vi "get_saved_XYZ_pos.vi"(11 "MotorSystem.lvclass input":refnum<class "MotorSystem.lvclass">) -> (2 "points":cluster{"X":dbl, "Y":dbl, "Z":dbl}[](array[cluster]), 3 "MotorSystem.lvclass output":refnum<class "MotorSystem.lvclass">)   [LabVIEW 2016, in "MotionControl_UFO_3DOF.lvlib" / "MotorSystem.lvclass"]
uses:
  <userlib>/MotionControl_UFO_3DOF/MotorSystem/MotorSystem.lvclass
  <userlib>/MotionControl_UFO_3DOF/MotorSystem/MotorSystem.lvclass/MotorSystem.ctl
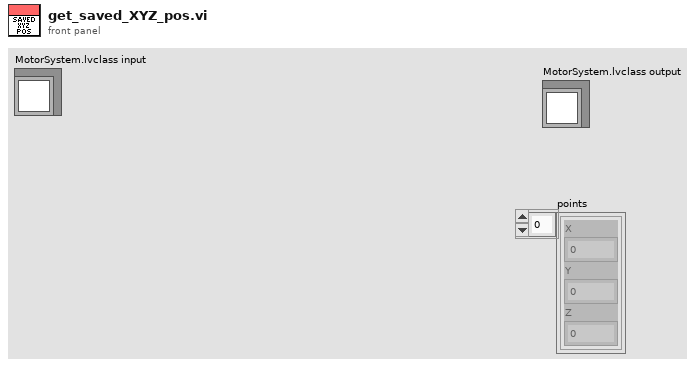
[diagram p1: front panel]
types:
  T1 = typedef "MotionControl_UFO_3DOF.lvlib/MotorSystem.lvclass/SavedPosCluster.ctl" = cluster{"name":string, "command list":T2}
  T2 = typedef "MotionControl_UFO_3DOF.lvlib/MotorSystem.lvclass/CommandList.ctl" = cluster{"cmd":T3, "cmd info":T4[]}[]
  T3 = typedef "MotionControl_UFO_3DOF.lvlib/MotorSystem.lvclass/cmd_system.ctl" = enum16{"NONE", "MOVE_SYSTEM", "WAIT_UNTIL_MOVE_DONE", "EXIT", "WAIT_UNTIL_SELECTED_MOVE_DONE", "WAIT_A_TIME"}
  T4 = typedef "MotionControl_UFO_3DOF.lvlib/MotorSystem.lvclass/SavedDimensionCluster.ctl" = cluster{"dimension name":string, "pos":dbl, "unit mode":T5, "unit conversion ratio":dbl}
  T5 = typedef "MotionControl_UFO_3DOF.lvlib/OneMotion.lvclass/unit mode.ctl" = enum16{"motor (pulse)", "linear (mm) or radial (degree)"}
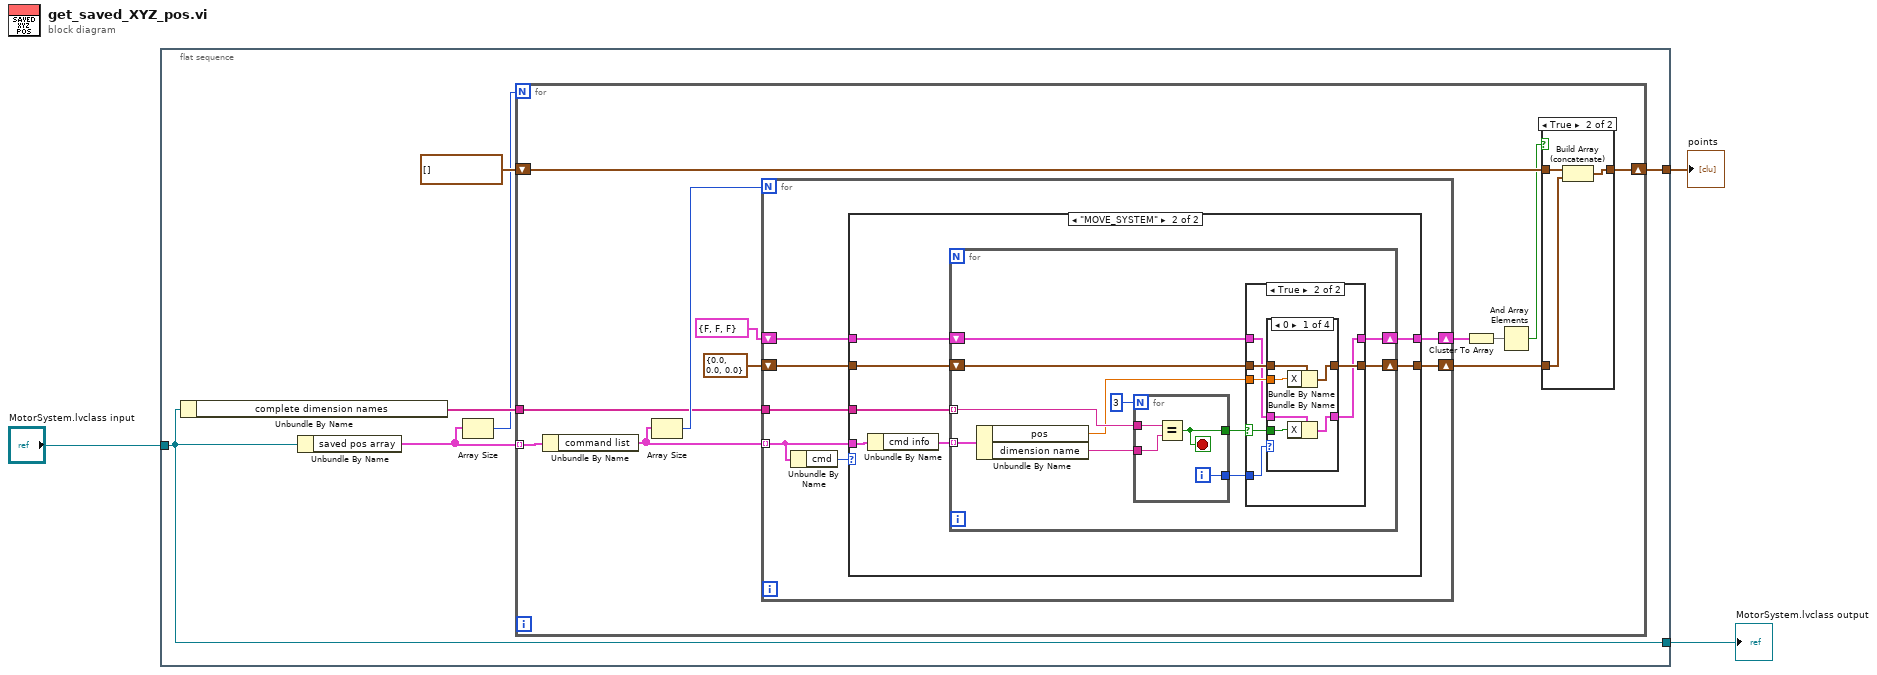
[diagram p0: block diagram]
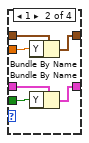
[diagram p5: hidden frame]
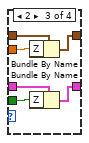
[diagram p6: hidden frame]
diagram:
  n1 = flat-sequence {
    tunnel: "MotorSystem.lvclass input" -> [w4]
    tunnel: [w4] -> w2
    tunnel: [w6] -> w1
    frame #0 {
      n2 = Unbundle By Name(w4) -> ("complete dimension names"=w9:string[])
      n3 = Unbundle By Name(w4) -> ("saved pos array"=w5:T1[])
      n4 = Array Size(array=w5) -> (size(s)=w7:i32)
      n5 = for {
        N: w7 -> [_]
        tunnel: w5 -> [w21] mode=indexing
        tunnel: w9 -> [w18]
        shift-right: [w14] -> w6
        shift-left: cluster{"X":dbl, "Y":dbl, "Z":dbl}[] [] ("points") -> [w16]
        n6 = Unbundle By Name(w21) -> ("command list"=w20:T2)
        n7 = Array Size(array=w20) -> (size(s)=w19:i32)
        n8 = for {
          N: w19 -> [_]
          tunnel: w20 -> [w27] mode=indexing
          tunnel: w18 -> [w32]
          shift-right: [w30] -> w15
          shift-left: cluster{"X":dbl, "Y":dbl, "Z":dbl} {"X"=0.0, "Y"=0.0, "Z"=0.0} ("target") -> [w31]
          shift-right: [w28] -> w12
          shift-left: cluster{"X":bool, "Y":bool, "Z":bool} {"X"=FALSE, "Y"=FALSE, "Z"=FALSE} -> [w29]
          n9 = Unbundle By Name(w27) -> ("cmd"=w26:T3)
          n10 = case shown="\"MOVE_SYSTEM\"" w26 {
            tunnel: w32 -> [_ w41]
            tunnel: w31 -> [w34 w40]
            tunnel: [w34 w39] -> w30
            tunnel: w29 -> [w33 w38]
            tunnel: [w33 w37] -> w28
            tunnel: w27 -> [_ w36]
            frame "NONE", Default {
            }
            frame "MOVE_SYSTEM" {
              n11 = Unbundle By Name(w36) -> ("cmd info"=w35:T4[])
              n12 = for {
                tunnel: w41 -> [w51] mode=indexing
                shift-right: [w47] -> w39
                shift-left: w40 -> [w49]
                shift-right: [w45] -> w37
                shift-left: w38 -> [w46]
                tunnel: w35 -> [w43] mode=indexing
                n13 = Unbundle By Name(w43) -> ("pos"=w48:dbl, "dimension name"=w42:string)
                n14 = for {
                  N: 3 -> [_]
                  tunnel: w51 -> [w85]
                  tunnel: w42 -> [w84]
                  tunnel: [w83] -> w50
                  tunnel: [w82] -> w44
                  i -> [w83]
                  stop <- w82 stop-if-true
                  n15 = Equal?(x=w85, y=w84) -> (x = y?=w82:bool)
                }
                n16 = case shown="True" w44 {
                  selector: w44 -> [_ w55]
                  tunnel: w50 -> [_ w61]
                  tunnel: w49 -> [w53 w60]
                  tunnel: w48 -> [_ w59]
                  tunnel: [w53 w58] -> w47
                  tunnel: w46 -> [w54 w57]
                  tunnel: [w54 w56] -> w45
                  frame False {
                  }
                  frame True {
                    n17 = case shown="0" w61 {
                      tunnel: w60 -> [w67 w73 w79 w81]
                      tunnel: w59 -> [w66 w72 w78 _]
                      tunnel: [w65 w71 w77 w81] -> w58
                      tunnel: w57 -> [w64 w70 w76 w80]
                      tunnel: [w62 w68 w74 w80] -> w56
                      tunnel: w55 -> [w63 w69 w75 _]
                      frame 0 {
                        n18 = Bundle By Name(cluster=w67, "X"=w66) -> (w65:cluster{"X":dbl, "Y":dbl, "Z":dbl})
                        n19 = Bundle By Name(cluster=w64, "X"=w63) -> (w62:cluster{"X":bool, "Y":bool, "Z":bool})
                      }
                      frame 1 {
                        n20 = Bundle By Name(cluster=w73, "Y"=w72) -> (w71:cluster{"X":dbl, "Y":dbl, "Z":dbl})
                        n21 = Bundle By Name(cluster=w70, "Y"=w69) -> (w68:cluster{"X":bool, "Y":bool, "Z":bool})
                      }
                      frame 2 {
                        n22 = Bundle By Name(cluster=w79, "Z"=w78) -> (w77:cluster{"X":dbl, "Y":dbl, "Z":dbl})
                        n23 = Bundle By Name(cluster=w76, "Z"=w75) -> (w74:cluster{"X":bool, "Y":bool, "Z":bool})
                      }
                      frame 3, Default {
                      }
                    }
                  }
                }
              }
            }
          }
        }
        n24 = Cluster To Array(cluster=w12) -> (array=w11:bool[])
        n25 = And Array Elements(Boolean array=w11) -> (logical AND=w10:bool)
        n26 = case shown="True" w10 {
          tunnel: w16 -> [w22 w25]
          tunnel: w15 -> [_ w24]
          tunnel: [w22 w23] -> w14
          frame False {
          }
          frame True {
            n27 = Build Array (concatenate)(w25, w24) -> (w23:cluster{"X":dbl, "Y":dbl, "Z":dbl}[])
          }
        }
      }
    }
  }
  "MotorSystem.lvclass output" <- w2
  "points" <- w1
